vi "GetGearManipulatorRelease.vi"() -> (2 "Gear Manipulator Release":bool)   [LabVIEW 2016, in "Gear Manipulator.lvclass"]
uses:
  Gear Manipulator.lvclass
  Gear Manipulator.lvclass/Gear Manipulator.ctl
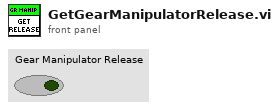
[diagram p1: front panel]
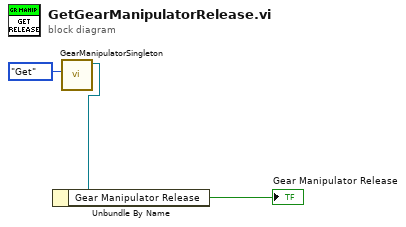
[diagram p0: block diagram]
diagram:
  n1 = call "GearManipulatorSingleton.vi"("Get/Set"=enum16{"Get", "Set"}."Get") -> ("Gear Manipulator.lvclass"=w1:refnum<class "Gear Manipulator.lvclass">)  [unwired: 9 in, 1 out]
  n2 = Unbundle By Name(w1) -> ("Gear Manipulator Release"=→"Gear Manipulator Release":bool)
